vi "DOCK_gear_status_number_to_description_and_enum.vi"(11 "status_nmb":string) -> (2 "status_enum":T1, 3 "status_description":string)   [LabVIEW 2019]
uses:
  DOCK_gear_statuses.ctl
  _misc/AULocalize/SubVIs/Get Localized Phrase Compact Interface 0D.vi
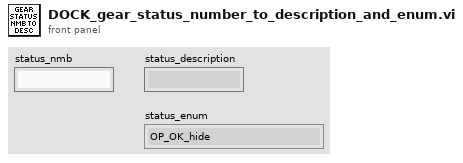
[diagram p1: front panel]
types:
  T1 = typedef "DOCK_GEAR_statuses.ctl" = enum16{"OP_OK_hide", "OP_OK_show", "OP_NOK_hide", "OP_NOK_show", "OP_interrupted_hide", "OP_interrupted_show", "OP_in_operation_hide", "OP_in_operation_show", "OP_unexpected_hide", "OP_unexpected_show", "RE_REAL_OK", "RE_REAL_NOK", "RE_STRING", "RE_sub_header", "RE_no_data", "RE_unexpected", "BA_sub_header", "BA_data", "BA_no_data"}
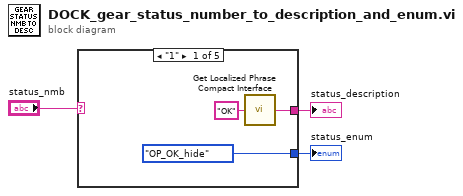
[diagram p0: block diagram]
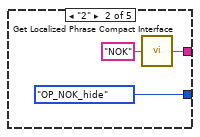
[diagram p2: hidden frame]
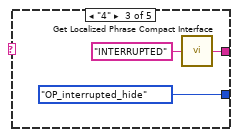
[diagram p3: hidden frame]
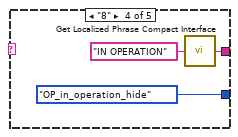
[diagram p4: hidden frame]
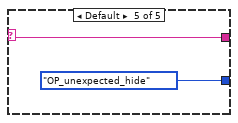
[diagram p5: hidden frame]
diagram:
  n1 = case shown="\"1\"" "status_nmb" {
    selector: "status_nmb" -> [_ _ _ _ w16]
    tunnel: [DOCK_GEAR_statuses."OP_OK_hide" ("REPORT_GEAR_statuses") DOCK_GEAR_statuses."OP_NOK_hide" ("REPORT_GEAR_statuses") DOCK_GEAR_statuses."OP_interrupted_hide" ("REPORT_GEAR_statuses") DOCK_GEAR_statuses."OP_in_operation_hide" ("REPORT_GEAR_statuses") DOCK_GEAR_statuses."OP_unexpected_hide" ("REPORT_GEAR_statuses")] -> w2
    tunnel: [w4 w7 w10 w13 w16] -> w3
    frame "1" {
      n2 = call-poly "Get Localized Phrase Compact Interface.vi"("Key"="OK") -> ("Translated Phrase"=w4:string)
    }
    frame "2" {
      n3 = call-poly "Get Localized Phrase Compact Interface.vi"("Key"="NOK") -> ("Translated Phrase"=w7:string)
    }
    frame "4" {
      n4 = call-poly "Get Localized Phrase Compact Interface.vi"("Key"="INTERRUPTED") -> ("Translated Phrase"=w10:string)
    }
    frame "8" {
      n5 = call-poly "Get Localized Phrase Compact Interface.vi"("Key"="IN OPERATION") -> ("Translated Phrase"=w13:string)
    }
    frame Default {
    }
  }
  "status_description" <- w3
  "status_enum" <- w2
